vi "UpcastingTest.vi"() -> (2 "NonUpcast Col array":refnum<class "Column.lvclass">[](array[class]))   [LabVIEW 2012]
uses:
  ColumnVIs/Column/Column.lvclass
  ColumnVIs/SingleValCol/SingleValCol.lvclass
  ColumnVIs/DigitalCol/DigitalCol.lvclass
  ColumnVIs/GroupCol/GroupCol.lvclass
  ColumnVIs/TriggerCol/TriggerCol.lvclass
  ColumnVIs/ModeCOl/ModeCol.lvclass
panel:
  out "Upcast Column Array":refnum<class "Column.lvclass">[](array[class])
  # "Turns out the act of wiring together siblings automatically upcasts them to the nearest common ancenstor!\nIf the Upcast Column Array isn't populated, go to the Block diagram (CTRL-E) and right click the Disable box and \"Enable this subdiagram.\""
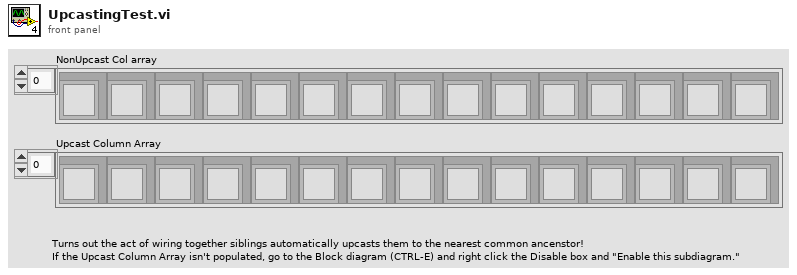
[diagram p1: front panel]
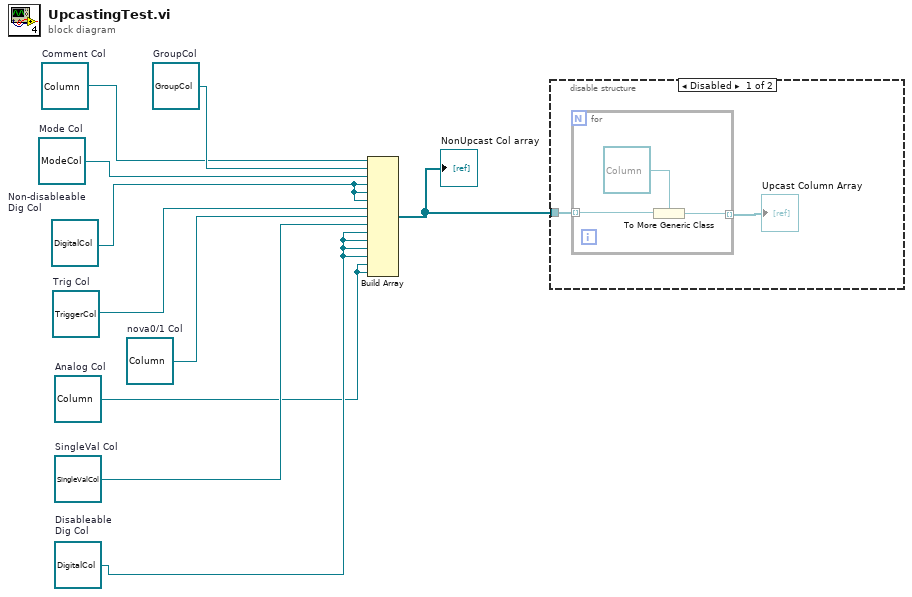
[diagram p0: block diagram]
diagram:
  w1 = refnum<class "ModeCol.lvclass"> refnum  # Mode Col
  w2 = refnum<class "TriggerCol.lvclass"> refnum  # Trig Col
  w3 = refnum<class "Column.lvclass"> refnum  # Comment Col
  w4 = refnum<class "GroupCol.lvclass"> refnum  # GroupCol
  w5 = refnum<class "Column.lvclass"> refnum  # Analog Col
  w6 = refnum<class "Column.lvclass"> refnum  # nova0/1 Col
  w7 = refnum<class "DigitalCol.lvclass"> refnum  # Disableable Dig Col
  w8 = refnum<class "DigitalCol.lvclass"> refnum  # Non-disableable  Dig Col
  w9 = refnum<class "SingleValCol.lvclass"> refnum  # SingleVal Col
  n1 = Build Array(w3, w4, w1, w8, w8, w8, w2, w6, w9, w7, w7, w7, w7, w5, w5) -> (w10:refnum<class "Column.lvclass">[])
  "NonUpcast Col array" <- w10
  n2 = disable-structure shown="Disabled" {
    disable-tunnel: w10 -> [w12 _]
    frame Disabled {
      n3 = for {
        tunnel: w12 -> [w15] mode=indexing
        tunnel: [w13] -> w11 mode=indexing
        n4 = To More Generic Class(target class=refnum<class "Column.lvclass"> refnum ("Column.lvclass"), reference=w15) -> (generic class reference=w13:refnum<class "Column.lvclass">)
      }
      "Upcast Column Array" <- w11
    }
    frame Enabled {
    }
  }
